vi "Sum Frame Images.vi"(8 "# Y Pixels":i64, 9 "# X Pixels":i64, 11 "Pixel Values":i32[](array[numeric])) -> (3 "Accumulated Image":i32[][](array[numeric]))   [LabVIEW 2021, in "PTU Files.lvlib"]
uses:
  PTU Files.lvlib
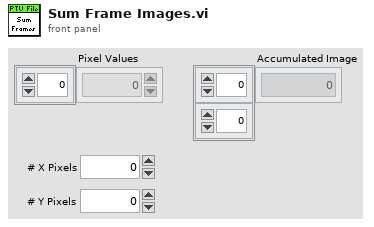
[diagram p1: front panel]
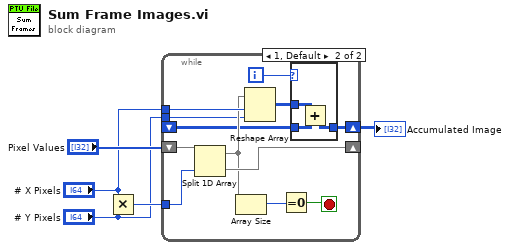
[diagram p0: block diagram]
diagram:
  n1 = Multiply(x="# X Pixels", y="# Y Pixels") -> (x*y=w4:i64)
  n2 = while {
    shift-right: [w15] -> _
    shift-left: "Pixel Values" -> [w17]
    tunnel: w4 -> [w16]
    tunnel: "# X Pixels" -> [w12]
    tunnel: "# Y Pixels" -> [w10]
    shift-right: [w8] -> w1
    shift-left: _ -> [w6]
    i -> [w9]
    stop <- w13 stop-if-true
    n3 = Split 1D Array(array=w17, index=w16) -> (first subarray=w11:i32[], second subarray=w15:i32[])
    n4 = Array Size(array=w11) -> (size(s)=w14:i32)
    n5 = Reshape Array(w11, w12, w10) -> (w7:i32[][])
    n6 = Equal To 0?(x=w14) -> (x = 0?=w13:bool)
    n7 = case shown="1, Default" w9 {
      tunnel: [w18 w19] -> w8
      tunnel: w7 -> [w18 w21]
      tunnel: w6 -> [_ w20]
      frame 0 {
      }
      frame 1, Default {
        n8 = Add(x=w21, y=w20) -> (x+y=w19:i32[][])
      }
    }
  }
  "Accumulated Image" <- w1
